vi "DriveVelocityHeadingFollower.vi"(0 "RobotMotors":T18={"DriveLeftPrimary"={"DeviceStatus"={"status"=FALSE, "code"=0, "source"=""}, "Type"=enum."PWM", "PWM"={"PWM Channel"=enum."PWM 1", "DeadBand"={"Name"="", "maxPositivePwm"=0, "minPositivePwm"=0, "centerPwm"=0, "maxNegativePwm"=0, "minNegativePwm"=0, "angularRange"=0}}, "CAN"={"Device Number"=0, "SetOutput VI Ref"=variant(enum8{"Percent VBus", "Current", "Speed", "Position", "Voltage"} enum."Percent VBus"), "GetOutput VI Ref"=variant(refnum<k1> refnum), "Enable VI Ref"=variant(dbl 12.0), "Disable VI Ref"=variant(enum8{"Percent VBus", "Speed", "Position", "Slave", "Unchanged / Invalid", "Voltage Compensation", "Current", "Motion Profile"} enum."Percent VBus"), "Data"=variant}, "Invert"=FALSE, "DIO PWM"={"PWM \"Enable\" Channel"=enum."Invalid", "DIOChannel"=enum."Invalid", "PWM Rate"=0.0}}, "DriveLeftSecondary1"={"DeviceStatus"={"status"=FALSE, "code"=0, "source"=""}, "Type"=enum."PWM", "PWM"={"PWM Channel"=enum."PWM 1", "DeadBand"={"Name"="", "maxPositivePwm"=0, "minPositivePwm"=0, "centerPwm"=0, "maxNegativePwm"=0, "minNegativePwm"=0, "angularRange"=0}}, "CAN"={"Device Number"=0, "SetOutput VI Ref"=variant(enum8{"Percent VBus", "Current", "Speed", "Position", "Voltage"} enum."Percent VBus"), "GetOutput VI Ref"=variant(refnum<k1> refnum), "Enable VI Ref"=variant(dbl 12.0), "Disable VI Ref"=variant(enum8{"Percent VBus", "Speed", "Position", "Slave", "Unchanged / Invalid", "Voltage Compensation", "Current", "Motion Profile"} enum."Percent VBus"), "Data"=variant}, "Invert"=FALSE, "DIO PWM"={"PWM \"Enable\" Channel"=enum."Invalid", "DIOChannel"=enum."Invalid", "PWM Rate"=0.0}}, "DriveRightPrimary"={"DeviceStatus"={"status"=FALSE, "code"=0, "source"=""}, "Type"=enum."PWM", "PWM"={"PWM Channel"=enum."PWM 1", "DeadBand"={"Name"="", "maxPositivePwm"=0, "minPositivePwm"=0, "centerPwm"=0, "maxNegativePwm"=0, "minNegativePwm"=0, "angularRange"=0}}, "CAN"={"Device Number"=0, "SetOutput VI Ref"=variant(enum8{"Percent VBus", "Current", "Speed", "Position", "Voltage"} enum."Percent VBus"), "GetOutput VI Ref"=variant(refnum<k1> refnum), "Enable VI Ref"=variant(dbl 12.0), "Disable VI Ref"=variant(enum8{"Percent VBus", "Speed", "Position", "Slave", "Unchanged / Invalid", "Voltage Compensation", "Current", "Motion Profile"} enum."Percent VBus"), "Data"=variant}, "Invert"=FALSE, "DIO PWM"={"PWM \"Enable\" Channel"=enum."Invalid", "DIOChannel"=enum."Invalid", "PWM Rate"=0.0}}, "DriveRightSecondary1"={"DeviceStatus"={"status"=FALSE, "code"=0, "source"=""}, "Type"=enum."PWM", "PWM"={"PWM Channel"=enum."PWM 1", "DeadBand"={"Name"="", "maxPositivePwm"=0, "minPositivePwm"=0, "centerPwm"=0, "maxNegativePwm"=0, "minNegativePwm"=0, "angularRange"=0}}, "CAN"={"Device Number"=0, "SetOutput VI Ref"=variant(enum8{"Percent VBus", "Current", "Speed", "Position", "Voltage"} enum."Percent VBus"), "GetOutput VI Ref"=variant(refnum<k1> refnum), "Enable VI Ref"=variant(dbl 12.0), "Disable VI Ref"=variant(enum8{"Percent VBus", "Speed", "Position", "Slave", "Unchanged / Invalid", "Voltage Compensation", "Current", "Motion Profile"} enum."Percent VBus"), "Data"=variant}, "Invert"=FALSE, "DIO PWM"={"PWM \"Enable\" Channel"=enum."Invalid", "DIOChannel"=enum."Invalid", "PWM Rate"=0.0}}, " RightIntake"={"DeviceStatus"={"status"=FALSE, "code"=0, "source"=""}, "Type"=enum."PWM", "PWM"={"PWM Channel"=enum."PWM 1", "DeadBand"={"Name"="", "maxPositivePwm"=0, "minPositivePwm"=0, "centerPwm"=0, "maxNegativePwm"=0, "minNegativePwm"=0, "angularRange"=0}}, "CAN"={"Device Number"=0, "SetOutput VI Ref"=variant(enum8{"Percent VBus", "Current", "Speed", "Position", "Voltage"} enum."Percent VBus"), "GetOutput VI Ref"=variant(refnum<k1> refnum), "Enable VI Ref"=variant(dbl 12.0), "Disable VI Ref"=variant(enum8{"Percent VBus", "Speed", "Position", "Slave", "Unchanged / Invalid", "Voltage Compensation", "Current", "Motion Profile"} enum."Percent VBus"), "Data"=variant}, "Invert"=FALSE, "DIO PWM"={"PWM \"Enable\" Channel"=enum."Invalid", "DIOChannel"=enum."Invalid", "PWM Rate"=0.0}}, "LeftIntake"={"DeviceStatus"={"status"=FALSE, "code"=0, "source"=""}, "Type"=enum."PWM", "PWM"={"PWM Channel"=enum."PWM 1", "DeadBand"={"Name"="", "maxPositivePwm"=0, "minPositivePwm"=0, "centerPwm"=0, "maxNegativePwm"=0, "minNegativePwm"=0, "angularRange"=0}}, "CAN"={"Device Number"=0, "SetOutput VI Ref"=variant(enum8{"Percent VBus", "Current", "Speed", "Position", "Voltage"} enum."Percent VBus"), "GetOutput VI Ref"=variant(refnum<k1> refnum), "Enable VI Ref"=variant(dbl 12.0), "Disable VI Ref"=variant(enum8{"Percent VBus", "Speed", "Position", "Slave", "Unchanged / Invalid", "Voltage Compensation", "Current", "Motion Profile"} enum."Percent VBus"), "Data"=variant}, "Invert"=FALSE, "DIO PWM"={"PWM \"Enable\" Channel"=enum."Invalid", "DIOChannel"=enum."Invalid", "PWM Rate"=0.0}}, "ArmPivot"={"DeviceStatus"={"status"=FALSE, "code"=0, "source"=""}, "Type"=enum."PWM", "PWM"={"PWM Channel"=enum."PWM 1", "DeadBand"={"Name"="", "maxPositivePwm"=0, "minPositivePwm"=0, "centerPwm"=0, "maxNegativePwm"=0, "minNegativePwm"=0, "angularRange"=0}}, "CAN"={"Device Number"=0, "SetOutput VI Ref"=variant(enum8{"Percent VBus", "Current", "Speed", "Position", "Voltage"} enum."Percent VBus"), "GetOutput VI Ref"=variant(refnum<k1> refnum), "Enable VI Ref"=variant(dbl 12.0), "Disable VI Ref"=variant(enum8{"Percent VBus", "Speed", "Position", "Slave", "Unchanged / Invalid", "Voltage Compensation", "Current", "Motion Profile"} enum."Percent VBus"), "Data"=variant}, "Invert"=FALSE, "DIO PWM"={"PWM \"Enable\" Channel"=enum."Invalid", "DIOChannel"=enum."Invalid", "PWM Rate"=0.0}}, "ArmPivot 2 "={"DeviceStatus"={"status"=FALSE, "code"=0, "source"=""}, "Type"=enum."PWM", "PWM"={"PWM Channel"=enum."PWM 1", "DeadBand"={"Name"="", "maxPositivePwm"=0, "minPositivePwm"=0, "centerPwm"=0, "maxNegativePwm"=0, "minNegativePwm"=0, "angularRange"=0}}, "CAN"={"Device Number"=0, "SetOutput VI Ref"=variant(enum8{"Percent VBus", "Current", "Speed", "Position", "Voltage"} enum."Percent VBus"), "GetOutput VI Ref"=variant(refnum<k1> refnum), "Enable VI Ref"=variant(dbl 12.0), "Disable VI Ref"=variant(enum8{"Percent VBus", "Speed", "Position", "Slave", "Unchanged / Invalid", "Voltage Compensation", "Current", "Motion Profile"} enum."Percent VBus"), "Data"=variant}, "Invert"=FALSE, "DIO PWM"={"PWM \"Enable\" Channel"=enum."Invalid", "DIOChannel"=enum."Invalid", "PWM Rate"=0.0}}, "ArmExtend "={"DeviceStatus"={"status"=FALSE, "code"=0, "source"=""}, "Type"=enum."PWM", "PWM"={"PWM Channel"=enum."PWM 1", "DeadBand"={"Name"="", "maxPositivePwm"=0, "minPositivePwm"=0, "centerPwm"=0, "maxNegativePwm"=0, "minNegativePwm"=0, "angularRange"=0}}, "CAN"={"Device Number"=0, "SetOutput VI Ref"=variant(enum8{"Percent VBus", "Current", "Speed", "Position", "Voltage"} enum."Percent VBus"), "GetOutput VI Ref"=variant(refnum<k1> refnum), "Enable VI Ref"=variant(dbl 12.0), "Disable VI Ref"=variant(enum8{"Percent VBus", "Speed", "Position", "Slave", "Unchanged / Invalid", "Voltage Compensation", "Current", "Motion Profile"} enum."Percent VBus"), "Data"=variant}, "Invert"=FALSE, "DIO PWM"={"PWM \"Enable\" Channel"=enum."Invalid", "DIOChannel"=enum."Invalid", "PWM Rate"=0.0}}, "Climber"={"DeviceStatus"={"status"=FALSE, "code"=0, "source"=""}, "Type"=enum."PWM", "PWM"={"PWM Channel"=enum."PWM 1", "DeadBand"={"Name"="", "maxPositivePwm"=0, "minPositivePwm"=0, "centerPwm"=0, "maxNegativePwm"=0, "minNegativePwm"=0, "angularRange"=0}}, "CAN"={"Device Number"=0, "SetOutput VI Ref"=variant(enum8{"Percent VBus", "Current", "Speed", "Position", "Voltage"} enum."Percent VBus"), "GetOutput VI Ref"=variant(refnum<k1> refnum), "Enable VI Ref"=variant(dbl 12.0), "Disable VI Ref"=variant(enum8{"Percent VBus", "Speed", "Position", "Slave", "Unchanged / Invalid", "Voltage Compensation", "Current", "Motion Profile"} enum."Percent VBus"), "Data"=variant}, "Invert"=FALSE, "DIO PWM"={"PWM \"Enable\" Channel"=enum."Invalid", "DIOChannel"=enum."Invalid", "PWM Rate"=0.0}}, "SelfieStick"={"DeviceStatus"={"status"=FALSE, "code"=0, "source"=""}, "Type"=enum."PWM", "PWM"={"PWM Channel"=enum."PWM 1", "DeadBand"={"Name"="", "maxPositivePwm"=0, "minPositivePwm"=0, "centerPwm"=0, "maxNegativePwm"=0, "minNegativePwm"=0, "angularRange"=0}}, "CAN"={"Device Number"=0, "SetOutput VI Ref"=variant(enum8{"Percent VBus", "Current", "Speed", "Position", "Voltage"} enum."Percent VBus"), "GetOutput VI Ref"=variant(refnum<k1> refnum), "Enable VI Ref"=variant(dbl 12.0), "Disable VI Ref"=variant(enum8{"Percent VBus", "Speed", "Position", "Slave", "Unchanged / Invalid", "Voltage Compensation", "Current", "Motion Profile"} enum."Percent VBus"), "Data"=variant}, "Invert"=FALSE, "DIO PWM"={"PWM \"Enable\" Channel"=enum."Invalid", "DIOChannel"=enum."Invalid", "PWM Rate"=0.0}}}, 1 "RobotConfig":T3={"Motors"={"DriveLeftPrimary"={"CAN Address"=1, "Invert"=FALSE, "InvertSensor"=FALSE, "Unit Conversion Factor"=0.0, "Brake Mode"=enum."Override to Brake", "Reverse Limt Switch Mode"=enum."Normally Closed", "Forward Limt Swith Mode"=enum."Normally Closed"}, "DriveLeftSecondary1"={"CAN Address"=2, "Invert"=FALSE, "InvertSensor"=FALSE, "Unit Conversion Factor"=0.0, "Brake Mode"=enum."Override to Brake", "Reverse Limt Switch Mode"=enum."Normally Closed", "Forward Limt Swith Mode"=enum."Normally Closed"}, "DriveRightPrimary"={"CAN Address"=3, "Invert"=FALSE, "InvertSensor"=FALSE, "Unit Conversion Factor"=0.0, "Brake Mode"=enum."Override to Brake", "Reverse Limt Switch Mode"=enum."Normally Closed", "Forward Limt Swith Mode"=enum."Normally Closed"}, "DriveRightSecondary1"={"CAN Address"=4, "Invert"=FALSE, "InvertSensor"=FALSE, "Unit Conversion Factor"=0.0, "Brake Mode"=enum."Override to Brake", "Reverse Limt Switch Mode"=enum."Normally Closed", "Forward Limt Swith Mode"=enum."Normally Closed"}, "RightIntake"={"CAN Address"=8, "Invert"=FALSE, "InvertSensor"=FALSE, "Unit Conversion Factor"=0.0, "Brake Mode"=enum."Override to Brake", "Reverse Limt Switch Mode"=enum."Normally Closed", "Forward Limt Swith Mode"=enum."Normally Closed"}, "LeftIntake"={"CAN Address"=7, "Invert"=FALSE, "InvertSensor"=FALSE, "Unit Conversion Factor"=0.0, "Brake Mode"=enum."Override to Brake", "Reverse Limt Switch Mode"=enum."Normally Closed", "Forward Limt Swith Mode"=enum."Normally Closed"}, "ArmPivot"={"CAN Address"=5, "Invert"=FALSE, "InvertSensor"=FALSE, "Unit Conversion Factor"=0.0, "Brake Mode"=enum."Override to Brake", "Reverse Limt Switch Mode"=enum."Normally Closed", "Forward Limt Swith Mode"=enum."Normally Closed"}, "ArmExtend"={"CAN Address"=6, "Invert"=FALSE, "InvertSensor"=FALSE, "Unit Conversion Factor"=0.0, "Brake Mode"=enum."Override to Brake", "Reverse Limt Switch Mode"=enum."Normally Closed", "Forward Limt Swith Mode"=enum."Normally Closed"}, "ArmPivot2"={"CAN Address"=9, "Invert"=FALSE, "InvertSensor"=FALSE, "Unit Conversion Factor"=0.0, "Brake Mode"=enum."Override to Brake", "Reverse Limt Switch Mode"=enum."Normally Closed", "Forward Limt Swith Mode"=enum."Normally Closed"}, "Climber"={"CAN Address"=10, "Invert"=FALSE, "InvertSensor"=FALSE, "Unit Conversion Factor"=0.0, "Brake Mode"=enum."Override to Brake", "Reverse Limt Switch Mode"=enum."Disabled", "Forward Limt Swith Mode"=enum."Disabled"}, "Selfie Stick"={"CAN Address"=11, "Invert"=FALSE, "InvertSensor"=FALSE, "Unit Conversion Factor"=0.0, "Brake Mode"=enum."Override to Brake", "Reverse Limt Switch Mode"=enum."Disabled", "Forward Limt Swith Mode"=enum."Disabled"}}, "Sensors"={"IMU"={"Yaw Axis"=enum."Z", "SPI Bus"=enum."SPI MXP", "AHRS Algorithm"=enum."Complementary", "Calibration Time (s)"=3.0, "Calibrate On Open"=TRUE}, "LimitSwitch1"={"DIOChannel"=enum."DIO 0", "Active Low"=FALSE}, "LimitSwitch2"={"DIOChannel"=enum."DIO 1", "Active Low"=FALSE}, "BeamBreak"={"DIOChannel"=enum."DIO 2", "Active Low"=FALSE}, "JeVois"={"Baud Rate"=9600, "Parity"=0, "Data Bits"=8, "Stop Bits"=10, "Termination Char (0xA = '\\n' = LF)"=10, "Enable Termination Char? (T)"=TRUE, "Flow Control"=0, "Timeout Value (ms)"=5000, "Serial Port"=enum."Onboard RS-232"}}, "PID"={"ArmExtend"={"P"=0.0, "I"=0.0, "D"=0.0, "F"=0.0, "IZone"=0.0}, "ArmRotate"={"P"=0.0, "I"=0.0, "D"=0.0, "F"=0.0, "IZone"=0.0}, "Drive"={"P"=0.0, "I"=0.0, "D"=0.0, "F"=0.0, "IZone"=0.0}, "DriveGyro Kp ((in/sec)/deg)"=0.0, "CameraPole"={"P"=0.0, "I"=0.0, "D"=0.0, "F"=0.0, "IZone"=0.0}}, "Solenoids"={"ArmClaw"={"Forward Channel"=enum."Solenoid 0", "Invert"=FALSE, "Reverse Channel"=enum."Solenoid 0"}, "IntakeExtend"={"Forward Channel"=enum."Solenoid 1", "Invert"=FALSE, "Reverse Channel"=enum."Solenoid 0"}, "IntakeOpen"={"Forward Channel"=enum."Solenoid 2", "Invert"=FALSE, "Reverse Channel"=enum."Solenoid 0"}, " Shifter"={"Forward Channel"=enum."Solenoid 3", "Invert"=FALSE, "Reverse Channel"=enum."Solenoid 0"}}, "RobotDimensions "={"Length"=0.0, "Height"=0.0, "HeightOfBumpers"=0.0, "DistanceFromFrameEdgeToPyramid "=0.0, "HeightOfFrameToIntake"=0.0, "EdgeOfFrameToOrigin"=0.0}, "ArmHomePosition"={"Angle (rad)"=0.0, "Radius (in)"=0.0}, "SelfieStickParams"={"Home Height (in)"=0.0, "CruiseVelocity"=0, "MaxAccel"=0, "Low Height (in)"=0.0, "High Height (in)"=0.0}} {"Sensors"."JeVois"."Flow Control" items=["None", "XON/XOFF", "RTS/CTS", "XON/XOFF & RTS/CTS", "DTR/DSR", "XON/XOFF & DTR/DSR"]; "Sensors"."JeVois"."Termination Char (0xA = '\\n' = LF)" format="%.0x"; "Sensors"."JeVois"."Stop Bits" items=["1.0"=10, "1.5"=15, "2.0"=20]; "Sensors"."JeVois"."Parity" items=["None", "Odd", "Even", "Mark", "Space"]}, 2 "IMU DevRef":T1={"DevStatus"={"status"=FALSE, "code"=0, "source"=""}, "Handle"=0, "SPI Bus"=enum."SPI On-Board, CS0", "Device Found"=FALSE, "Device Ready"=FALSE, "Yaw Axis"=enum."Z", "AHRS Algorithm"=enum."Complementary", "Serial"=0, "Lot ID 2"=0, "Lot ID 1"=0, "Bytes Per Sample"=0, "Calibrate On Open?"=FALSE}, 3 "DriveCompleteNotifier":refnum<notifier>, 4 "DriveGyro Kp ((in/sec)/deg)":dbl) -> ()   [LabVIEW 2017]
uses:
  TypeDefs/RobotComponents/RobotMotors.ctl
  <vilib>/Rock Robotics/WPI/MotorControl/WPI_MotorControlDeviceRef.ctl
  <vilib>/Rock Robotics/WPI/MotorControl/WPI_MotorControlType.ctl
  <vilib>/Rock Robotics/SystemInterfaces/DIO/FPGA_DIOPWMChannel.ctl
  <vilib>/Rock Robotics/WPI/PWM/WPI_PWMDeadband.ctl
  <vilib>/Rock Robotics/SystemInterfaces/DIO/FPGA_DIOChannel.ctl
  TypeDefs/ConfigComponents/Config_Robot.ctl
  TypeDefs/ConfigComponents/Config_Motor.ctl
  <vilib>/Rock Robotics/WPI/ThirdParty/Phoenix-LabVIEW/Motor Controller/Controls/CTRE_Phoenix_MotorControl_NeutralMode.ctl
  <vilib>/Rock Robotics/WPI/ThirdParty/Phoenix-LabVIEW/Motor Controller/Controls/CTRE_Phoenix_MotorControl_LimitSwitchNormal.ctl
  TypeDefs/ConfigComponents/Config_IMU.ctl
  <vilib>/Rock Robotics/SystemInterfaces/spilib/spi_bus.ctl
  TypeDefs/ConfigComponents/Config_DigitalIO.ctl
  TypeDefs/ConfigComponents/Config_SerialPort.ctl
  <vilib>/Rock Robotics/WPI/SerialPort/WPI_SerialPort.ctl
  TypeDefs/ConfigComponents/Config_PIDParams.ctl
  TypeDefs/ConfigComponents/Config_DoubleSolenoid.ctl
  <vilib>/Rock Robotics/WPI/Solenoid/WPI_SolenoidChannel.ctl
  TypeDefs/ConfigComponents/Config_Dimensions.ctl
  TypeDefs/ConfigComponents/Config_ArmHome.ctl
  TypeDefs/ConfigComponents/Config_SelfieStick.ctl
  Sensors/IMU/ADI_IMU_ADIS16448_IMUDevRef.ctl
  ArgosLib/Signal Processing/TypeDefs/EdgeDetector_Type.ctl
  <vilib>/Rock Robotics/WPI/ThirdParty/Phoenix-LabVIEW/Motor Controller/Controls/CTRE_Phoenix_MotorControl_ControlMode.ctl
  Global_Var-RefNum/MotionProfileControlData.vi
  Sensors/IMU/ADIS16448_IMU.lvlib
  ArgosLib/ArgosLib.lvlib
panel:
  in  "MinCompletionPercent":dbl=0.5
  in  "Stopped Velocity Threshold (in/sec)":dbl=1.0
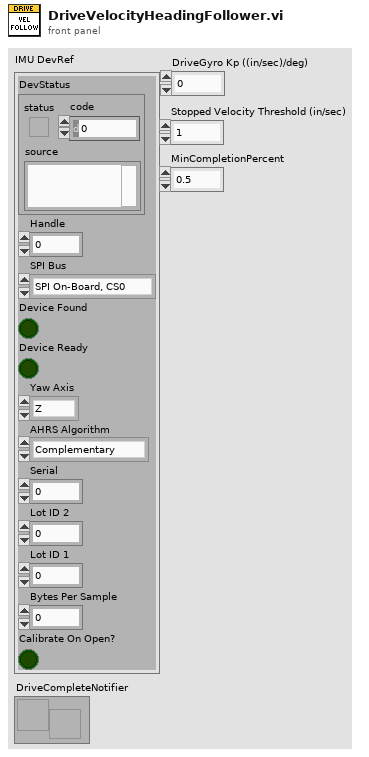
[diagram p1: front panel]
types:
  T1 = typedef "ADIS16448_IMU.lvlib/ADI_IMU_ADIS16448_IMUDevRef.ctl" = cluster{"DevStatus":errorcluster, "Handle":i32, "SPI Bus":T2, "Device Found":bool, "Device Ready":bool, "Yaw Axis":enum16{"X", "Y", "Z"}, "AHRS Algorithm":enum16{"Complementary", "Madgwick"}, "Serial":u16, "Lot ID 2":u16, "Lot ID 1":u16, "Bytes Per Sample":u16, "Calibrate On Open?":bool}
  T2 = typedef "spi_bus.ctl" = enum16{"SPI On-Board, CS0", "SPI On-Board, CS1", "SPI On-Board, CS2", "SPI On-Board, CS3", "SPI MXP", "Invalid"}
  T3 = typedef "Config_Robot.ctl" = cluster{"Motors":cluster{"DriveLeftPrimary":T4, "DriveLeftSecondary1":T4, "DriveRightPrimary":T4, "DriveRightSecondary1":T4, "RightIntake":T4, "LeftIntake":T4, "ArmPivot":T4, "ArmExtend":T4, "ArmPivot2":T4, "Climber":T4, "Selfie Stick":T4}, "Sensors":cluster{"IMU":T7, "LimitSwitch1":T8, "LimitSwitch2":T8, "BeamBreak":T8, "JeVois":T10}, "PID":cluster{"ArmExtend":T12, "ArmRotate":T12, "Drive":T12, "DriveGyro Kp ((in/sec)/deg)":dbl, "CameraPole":T12}, "Solenoids":cluster{"ArmClaw":T13, "IntakeExtend":T13, "IntakeOpen":T13, " Shifter":T13}, "RobotDimensions ":T15, "ArmHomePosition":T16, "SelfieStickParams":T17}
  T4 = typedef "Config_Motor.ctl" = cluster{"CAN Address":u8, "Invert":bool, "InvertSensor":bool, "Unit Conversion Factor":dbl, "Brake Mode":T5, "Reverse Limt Switch Mode":T6, "Forward Limt Swith Mode":T6}
  T5 = typedef "CTRE_Phoenix_MotorControl_NeutralMode.ctl" = enum8{"EEPROMSetting", "Override to Coast", "Override to Brake"}
  T6 = typedef "CTRE_Phoenix_MotorControl_LimitSwitchNormal.ctl" = enum16{"Normally Open", "Normally Closed", "Disabled"}
  T7 = typedef "Config_IMU.ctl" = cluster{"Yaw Axis":enum16{"X", "Y", "Z"}, "SPI Bus":T2, "AHRS Algorithm":enum16{"Complementary", "Madgwick"}, "Calibration Time (s)":dbl, "Calibrate On Open":bool}
  T8 = typedef "Config_DigitalIO.ctl" = cluster{"DIOChannel":T9, "Active Low":bool}
  T9 = typedef "FPGA_DIOChannel.ctl" = enum8{"DIO 0", "DIO 1", "DIO 2", "DIO 3", "DIO 4", "DIO 5", "DIO 6", "DIO 7", "DIO 8", "DIO 9", "DIO MXP 0", "DIO MXP 1", "DIO MXP 2", "DIO MXP 3", "DIO MXP 4", "DIO MXP 5", "DIO MXP 6", "DIO MXP 7", "DIO MXP 8", "DIO MXP 9", "DIO MXP 10", "DIO MXP 11", "DIO MXP 12", "DIO MXP 13", "DIO MXP 14", "DIO MXP 15", "SPI Port CS1", "SPI Port CS2", "SPI Port CS3", "SPI Port MISO", "SPI Port MOSI", "Invalid"}
  T10 = typedef "Config_SerialPort.ctl" = cluster{"Baud Rate":u32, "Parity":u16, "Data Bits":u16, "Stop Bits":u16, "Termination Char (0xA = '\\n' = LF)":u8, "Enable Termination Char? (T)":bool, "Flow Control":u16, "Timeout Value (ms)":u32, "Serial Port":T11}
  T11 = typedef "WPI_SerialPort.ctl" = enum16{"Onboard RS-232", "MXP TTL", "USB 1", "USB 2"}
  T12 = typedef "Config_PIDParams.ctl" = cluster{"P":dbl, "I":dbl, "D":dbl, "F":dbl, "IZone":dbl}
  T13 = typedef "Config_DoubleSolenoid.ctl" = cluster{"Forward Channel":T14, "Invert":bool, "Reverse Channel":T14}
  T14 = typedef "WPI_SolenoidChannel.ctl" = enum8{"Solenoid 0", "Solenoid 1", "Solenoid 2", "Solenoid 3", "Solenoid 4", "Solenoid 5", "Solenoid 6", "Solenoid 7", "Invalid"}
  T15 = typedef "Config_Dimensions.ctl" = cluster{"Length":dbl, "Height":dbl, "HeightOfBumpers":dbl, "DistanceFromFrameEdgeToPyramid ":dbl, "HeightOfFrameToIntake":dbl, "EdgeOfFrameToOrigin":dbl}
  T16 = typedef "Config_ArmHome.ctl" = cluster{"Angle (rad)":dbl, "Radius (in)":dbl}
  T17 = typedef "Config_SelfieStick.ctl" = cluster{"Home Height (in)":dbl, "CruiseVelocity":i32, "MaxAccel":i32, "Low Height (in)":dbl, "High Height (in)":dbl}
  T18 = typedef "RobotMotors.ctl" = cluster{"DriveLeftPrimary":T19, "DriveLeftSecondary1":T19, "DriveRightPrimary":T19, "DriveRightSecondary1":T19, " RightIntake":T19, "LeftIntake":T19, "ArmPivot":T19, "ArmPivot 2 ":T19, "ArmExtend ":T19, "Climber":T19, "SelfieStick":T19}
  T19 = typedef "WPI_MotorControlDeviceRef.ctl" = cluster{"DeviceStatus":errorcluster, "Type":T20, "PWM":cluster{"PWM Channel":T21, "DeadBand":T22}, "CAN":cluster{"Device Number":u8, "SetOutput VI Ref":variant, "GetOutput VI Ref":variant, "Enable VI Ref":variant, "Disable VI Ref":variant, "Data":variant}, "Invert":bool, "DIO PWM":cluster{"PWM \"Enable\" Channel":T21, "DIOChannel":T9, "PWM Rate":dbl}}
  T20 = typedef "WPI_MotorControlType.ctl" = enum16{"PWM", "CAN", "DIO PWM"}
  T21 = typedef "FPGA_DIOPWMChannel.ctl" = enum8{"PWM 0", "PWM 1", "PWM 2", "PWM 3", "PWM 4", "PWM 5", "PWM 6", "PWM 7", "PWM 8", "PWM 9", "PWM MXP 0", "PWM MXP 1", "PWM MXP 2", "PWM MXP 3", "PWM MXP 4", "PWM MXP 5", "PWM MXP 6", "PWM MXP 7", "PWM MXP 8", "PWM MXP 9", "Invalid"}
  T22 = typedef "WPI_PWMDeadband.ctl" = cluster{"Name":string, "maxPositivePwm":i32, "minPositivePwm":i32, "centerPwm":i32, "maxNegativePwm":i32, "minNegativePwm":i32, "angularRange":u16}
  T23 = typedef "ArgosLib.lvlib/EdgeDetector_Type.ctl" = enum16{"RisingEdge", "FallingEdge", "Both"}
  T24 = typedef "DriveMotionProfileControl.ctl" = cluster{"ControlMutex":T25, "Trajectory Points":T26[], "CurrentIndex":u32}
  T25 = typedef "Semaphore RefNum" = refnum<k1>
  T26 = typedef "Pathfinder.lvlib/Segment.ctl" = cluster{"dt":dbl, "x":dbl, "y":dbl, "position":dbl, "velocity":dbl, "acceleration":dbl, "jerk":dbl, "heading":dbl}
  T27 = cluster{"X Angle":dbl, "Y Angle":dbl, "Z Angle":dbl}
  T28 = typedef "CTRE_Phoenix_MotorControl_ControlMode.ctl" = u16
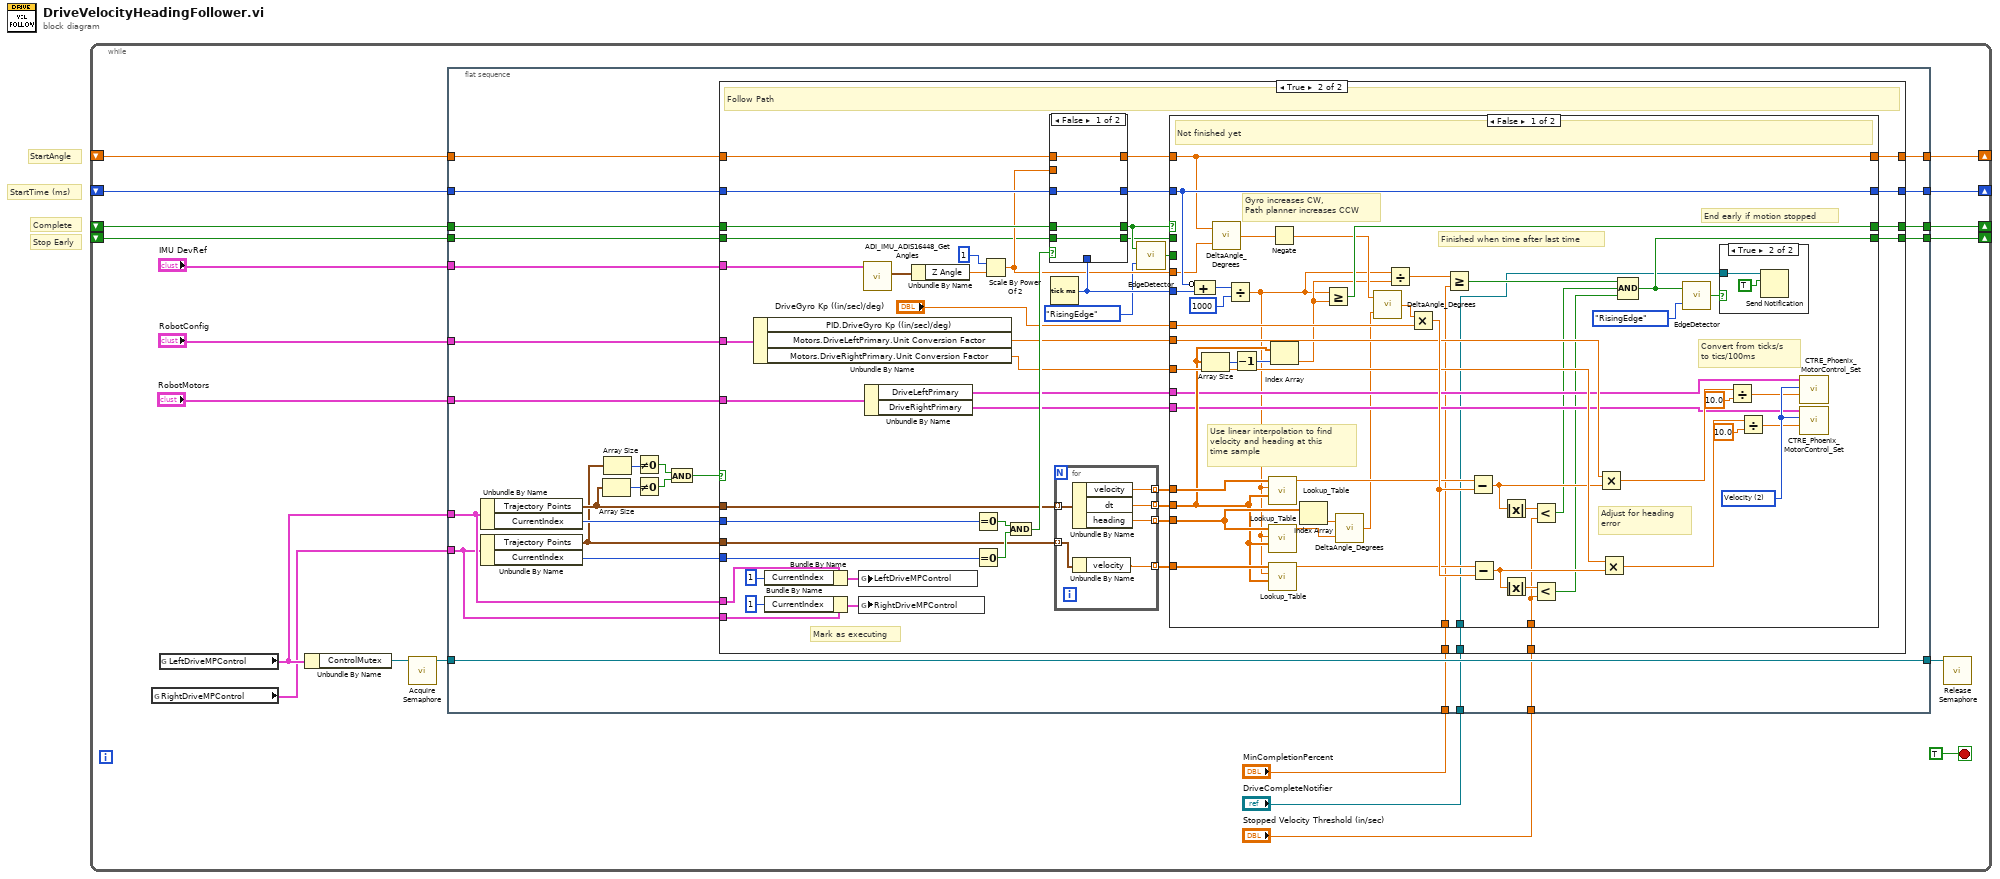
[diagram p0: block diagram]
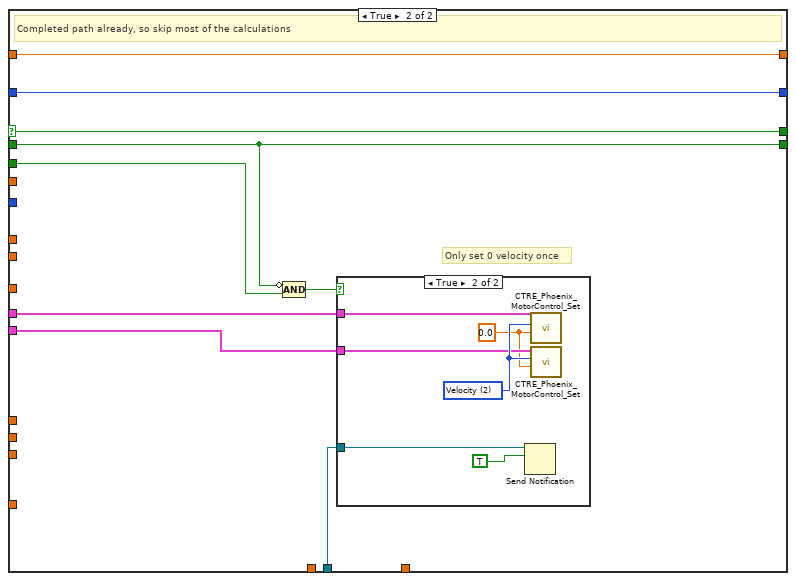
[diagram p4: hidden frame]
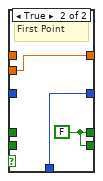
[diagram p6: hidden frame]
diagram:
  # "Stop Early"
  # "Complete"
  # "StartAngle"
  # "StartTime (ms)"
  n1 = while {
    shift-right: [w10] -> _
    shift-left: _ -> [w11]
    shift-right: [w9] -> _
    shift-left: _ -> [w8]
    shift-right: [w6] -> _
    shift-left: _ -> [w7]
    shift-right: [w5] -> _
    shift-left: _ -> [w4]
    stop <- TRUE stop-if-true
    n2 = global read "MotionProfileControlData.vi" "RightDriveMPControl"() -> (w16:T24)
    n3 = global read "MotionProfileControlData.vi" "LeftDriveMPControl"() -> (w17:T24)
    n4 = Unbundle By Name(w17) -> ("ControlMutex"=w20:T25)
    n5 = call <vilib>:"Acquire Semaphore.vi"("semaphore"=w20) -> ("semaphore out"=w19:T25)  [unwired: 4 in, 2 out]
    n6 = flat-sequence {
      tunnel: w19 -> [w46]
      tunnel: [w46] -> w18
      tunnel: w17 -> [w27]
      tunnel: w16 -> [w26]
      tunnel: "IMU DevRef" -> [w45]
      tunnel: "RobotMotors" -> [w44]
      tunnel: "RobotConfig" -> [w43]
      tunnel: w11 -> [w40]
      tunnel: [w37] -> w10
      tunnel: [w38] -> w9
      tunnel: w8 -> [w39]
      tunnel: w7 -> [w29]
      tunnel: [w28] -> w6
      tunnel: [w25] -> w5
      tunnel: w4 -> [w24]
      tunnel: "DriveCompleteNotifier" -> [w23]
      tunnel: "Stopped Velocity Threshold (in/sec)" -> [w22]
      tunnel: "MinCompletionPercent" -> [w21]
      frame #0 {
        n7 = Unbundle By Name(w27) -> ("Trajectory Points"=w36:T26[], "CurrentIndex"=w42:u32)
        n8 = Unbundle By Name(w26) -> ("Trajectory Points"=w35:T26[], "CurrentIndex"=w41:u32)
        n9 = Array Size(array=w36) -> (size(s)=w33:i32)
        n10 = Array Size(array=w35) -> (size(s)=w34:i32)
        n11 = Not Equal To 0?(x=w34) -> (x != 0?=w31:bool)
        n12 = Not Equal To 0?(x=w33) -> (x != 0?=w32:bool)
        n13 = And(x=w31, y=w32) -> (x .and. y?=w30:bool)
        n14 = case shown="True" w30 {
          tunnel: w45 -> [_ w96]
          tunnel: w44 -> [_ w95]
          tunnel: w43 -> [_ w94]
          tunnel: w42 -> [_ w93]
          tunnel: w41 -> [_ w92]
          tunnel: w40 -> [w49 w88]
          tunnel: w39 -> [w50 w87]
          tunnel: [w50 w77] -> w38
          tunnel: [w49 w75] -> w37
          tunnel: w36 -> [_ w81]
          tunnel: w35 -> [_ w80]
          tunnel: w29 -> [w48 w79]
          tunnel: [w48 w74] -> w28
          tunnel: w27 -> [_ w69]
          tunnel: w26 -> [_ w70]
          tunnel: [w47 w56] -> w25
          tunnel: w24 -> [w47 w54]
          tunnel: w23 -> [_ w53]
          tunnel: w22 -> [_ w52]
          tunnel: w21 -> [_ w51]
          frame False {
            # "No path to follow"
          }
          frame True {
            # "Mark as executing"
            # "Follow Path"
            n15 = Unbundle By Name(w94) -> ("Motors.DriveLeftPrimary.Unit Conversion Factor"=w64:dbl, "Motors.DriveRightPrimary.Unit Conversion Factor"=w63:dbl)  [unwired: 1 out]
            n16 = Bundle By Name(cluster=w69, "CurrentIndex"=u32 1) -> (w66:T24)
            n17 = Bundle By Name(cluster=w70, "CurrentIndex"=u32 1) -> (w65:T24)
            n18 = global write "MotionProfileControlData.vi" "LeftDriveMPControl"(w66) -> ()
            n19 = global write "MotionProfileControlData.vi" "RightDriveMPControl"(w65) -> ()
            n20 = call "ADI_IMU_ADIS16448_Get Angles.vi"("ADI IMU DevRef"=w96) -> ("IMU Angles Out"=w97:T27)  [unwired: 7 in, 3 out]
            n21 = Unbundle By Name(w95) -> ("DriveLeftPrimary"=w72:T19, "DriveRightPrimary"=w71:T19)
            n22 = Unbundle By Name(w97) -> ("Z Angle"=w86:dbl)
            n23 = Equal To 0?(x=w93) -> (x = 0?=w90:bool)
            n24 = Equal To 0?(x=w92) -> (x = 0?=w91:bool)
            n25 = Scale By Power Of 2(n=i16 1, x=w86) -> (x*2^n=w62:dbl)
            n26 = And(x=w90, y=w91) -> (x .and. y?=w89:bool)
            n27 = Tick Count (ms)() -> (millisecond timer value=w73:u32)
            n28 = case shown="False" w89 {
              tunnel: [w174 w176] -> w76
              tunnel: w88 -> [w174 _]
              tunnel: w62 -> [_ w177]
              tunnel: [w173 w177] -> w78
              tunnel: w87 -> [w173 _]
              tunnel: [w172 w175] -> w60
              tunnel: w79 -> [w172 _]
              tunnel: w73 -> [_ w176]
              tunnel: [w171 w175] -> w55
              tunnel: w54 -> [w171 _]
              frame False {
              }
              frame True {
                w175 = FALSE
                # "First Point"
              }
            }
            n29 = for {
              tunnel: w81 -> [w170] mode=indexing
              tunnel: w80 -> [w169] mode=indexing
              tunnel: [w168] -> w82 mode=indexing
              tunnel: [w167] -> w83 mode=indexing
              tunnel: [w166] -> w84 mode=indexing
              tunnel: [w165] -> w85 mode=indexing
              n30 = Unbundle By Name(w170) -> ("velocity"=w168:dbl, "dt"=w167:dbl, "heading"=w166:dbl)
              n31 = Unbundle By Name(w169) -> ("velocity"=w165:dbl)
            }
            n32 = call "EdgeDetector.vi"("DetectorType"=EdgeDetector_Type."RisingEdge", "Input"=w60) -> ("Edge"=w58:bool)
            n33 = case shown="False" w60 {
              selector: w60 -> [_ w156]
              tunnel: w62 -> [w119 _]
              tunnel: w73 -> [w147 _]
              tunnel: w85 -> [w145 _]
              tunnel: w84 -> [w142 _]
              tunnel: w83 -> [w131 _]
              tunnel: w82 -> [w144 _]
              tunnel: [w120 w157] -> w77
              tunnel: w78 -> [w120 w157]
              tunnel: w76 -> [w143 w158]
              tunnel: [w143 w158] -> w75
              tunnel: [w130 w156] -> w74
              tunnel: w72 -> [w128 w155]
              tunnel: w71 -> [w126 w154]
              tunnel: "DriveGyro Kp ((in/sec)/deg)" -> [w140 _]
              tunnel: w64 -> [w138 _]
              tunnel: w63 -> [w137 _]
              tunnel: w58 -> [_ w151]
              tunnel: [w103 w150] -> w56
              tunnel: w55 -> [_ w150]
              tunnel: w53 -> [w101 w153]
              tunnel: w52 -> [w109 _]
              tunnel: w51 -> [w105 _]
              frame False {
                w129 = T28 2 items=["PercentOutput"=0, "Position"=1, "Velocity"=2, "Current"=3, "Follower"=5, "MotionProfile"=6, "MotionMagic"=7, "MotionMagicArc"=8, "MotionProfileArc"=10, "Disabled"=15] ("Control Mode")
                # "End early if motion stopped"
                # "Gyro increases CW,\nPath planner increases CCW"
                # "Convert from ticks/s\nto tics/100ms"
                # "Adjust for heading\nerror"
                # "Use linear interpolation to find\nvelocity and heading at this\ntime sample"
                # "Finished when time after last time"
                # "Not finished yet"
                n34 = Compound Arithmetic op=ADD(invert w143, w147) -> (w134:u32)
                n35 = Array Size(array=w131) -> (size(s)=w133:i32)
                n36 = call "DeltaAngle_Degrees.vi"("EndAngle (deg)"=w119, "StartAngle (deg)"=w120) -> ("DeltaAngle (deg)"=w116:dbl)
                n37 = Divide(x=w134, y=u32 1000) -> (x/y=w98:dbl)
                n38 = Decrement(x=w133) -> (x-1=w132:i32)
                n39 = call "Lookup_Table.vi"("Y_Array"=w144, "x_in"=w98, "X_Array"=w131) -> ("y_out"=w136:dbl)  [unwired: 6 in]
                n40 = call "Lookup_Table.vi"("Y_Array"=w142, "x_in"=w98, "X_Array"=w131) -> ("y_out"=w117:dbl)  [unwired: 6 in]
                n41 = call "Lookup_Table.vi"("Y_Array"=w145, "x_in"=w98, "X_Array"=w131) -> ("y_out"=w135:dbl)  [unwired: 6 in]
                n42 = Negate(x=w116) -> (-x=w114:dbl)
                n43 = Index Array(array=w131, index=w132) -> (element=w99:dbl)
                n44 = Index Array(array=w142) -> (element=w118:dbl)  [unwired: 1 in]
                n45 = Greater Or Equal?(x=w98, y=w99) -> (x >= y?=w130:bool)
                n46 = call "DeltaAngle_Degrees.vi"("EndAngle (deg)"=w117, "StartAngle (deg)"=w118) -> ("DeltaAngle (deg)"=w115:dbl)
                n47 = call "DeltaAngle_Degrees.vi"("EndAngle (deg)"=w115, "StartAngle (deg)"=w114) -> ("DeltaAngle (deg)"=w141:dbl)
                n48 = Divide(x=w98, y=w99) -> (x/y=w106:dbl)
                n49 = Multiply(x=w141, y=w140) -> (x*y=w139:dbl)
                n50 = Greater Or Equal?(x=w106, y=w105) -> (x >= y?=w104:bool)
                n51 = Subtract(x=w136, y=w139) -> (x-y=w113:dbl)
                n52 = Subtract(x=w135, y=w139) -> (x-y=w110:dbl)
                n53 = Absolute Value(x=w113) -> (abs(x)=w112:dbl)
                n54 = Absolute Value(x=w110) -> (abs(x)=w111:dbl)
                n55 = Less?(x=w112, y=w109) -> (x < y?=w107:bool)
                n56 = Less?(x=w111, y=w109) -> (x < y?=w108:bool)
                n57 = Multiply(x=w138, y=w113) -> (x*y=w127:dbl)
                n58 = Multiply(x=w137, y=w110) -> (x*y=w125:dbl)
                n59 = Compound Arithmetic op=AND(w104, w107, w108) -> (w103:bool)
                n60 = call "EdgeDetector.vi"("DetectorType"=EdgeDetector_Type."RisingEdge", "Input"=w103) -> ("Edge"=w100:bool)
                n61 = case shown="True" w100 {
                  tunnel: w101 -> [_ w148]
                  frame False {
                  }
                  frame True {
                    n62 = Send Notification(notification=TRUE, notifier=w148) -> ()  [unwired: 1 in, 2 out]
                  }
                }
                n63 = Divide(x=w127, y=10.0) -> (x/y=w124:dbl)
                n64 = Divide(x=w125, y=10.0) -> (x/y=w122:dbl)
                n65 = call <vilib>:"CTRE_Phoenix_MotorControl_Set.vi"("Output"=w124, "Control Mode"=w129, "PhoenixMotorControlDevRef"=w128) -> ()  [unwired: 7 in, 2 out]
                n66 = call <vilib>:"CTRE_Phoenix_MotorControl_Set.vi"("Output"=w122, "Control Mode"=w129, "PhoenixMotorControlDevRef"=w126) -> ()  [unwired: 7 in, 2 out]
              }
              frame True {
                # "Only set 0 velocity once"
                # "Completed path already, so skip most of the calculations"
                n67 = Compound Arithmetic op=AND(invert w150, w151) -> (w152:bool)
                n68 = case shown="True" w152 {
                  tunnel: w155 -> [_ w163]
                  tunnel: w154 -> [_ w162]
                  tunnel: w153 -> [_ w159]
                  frame False {
                  }
                  frame True {
                    w161 = 0.0 ("Output")
                    w164 = T28 2 items=["PercentOutput"=0, "Position"=1, "Velocity"=2, "Current"=3, "Follower"=5, "MotionProfile"=6, "MotionMagic"=7, "MotionMagicArc"=8, "MotionProfileArc"=10, "Disabled"=15] ("Control Mode")
                    n69 = Send Notification(notification=TRUE, notifier=w159) -> ()  [unwired: 1 in, 2 out]
                    n70 = call <vilib>:"CTRE_Phoenix_MotorControl_Set.vi"("Output"=w161, "Control Mode"=w164, "PhoenixMotorControlDevRef"=w163) -> ()  [unwired: 7 in, 2 out]
                    n71 = call <vilib>:"CTRE_Phoenix_MotorControl_Set.vi"("Output"=w161, "Control Mode"=w164, "PhoenixMotorControlDevRef"=w162) -> ()  [unwired: 7 in, 2 out]
                  }
                }
              }
            }
          }
        }
      }
    }
    n72 = call <vilib>:"Release Semaphore.vi"("semaphore"=w18) -> ()  [unwired: 5 in, 2 out]
  }
